vi "domeADB_getEvent_BrakeEngaged.vi"(8 "error in (no error)":errorcluster, 11 "logevent_BrakeEngaged_Ctl":T1) -> (0 "error out":errorcluster, 2 "function return":i32, 3 "logevent_BrakeEngaged_Ctl out":T1)   [LabVIEW 2016, in "SALLV_domeADB.lvlib"]
doc: "int domeADB_shm_getEvent_BrakeEngagedLV(domeADB_logevent_BrakeEngagedLV *logevent_BrakeEngaged_Ctl );"
uses:
  SALLV_domeADB.lvlib
  DataTypes/logevent_BrakeEngaged.ctl
  SALLV_domeADB.so
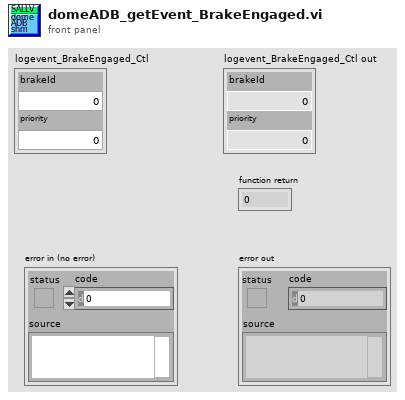
[diagram p1: front panel]
types:
  T1 = typedef "SALLV_domeADB.lvlib/logevent_BrakeEngaged.ctl" = cluster{"brakeId":i32, "priority":i32}
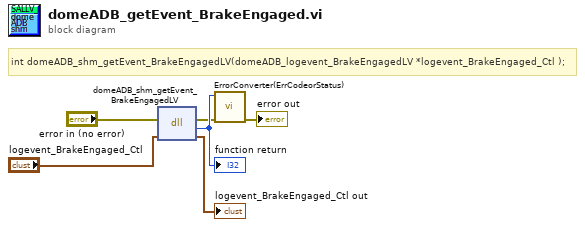
[diagram p0: block diagram]
diagram:
  # "int domeADB_shm_getEvent_BrakeEngagedLV(domeADB_logevent_BrakeEngagedLV *logevent_BrakeEngaged_Ctl );"
  n1 = dll-call lib="home/andres/Desktop/SALLV_domeADB/SALLV_domeADB.*" fn="domeADB_shm_getEvent_BrakeEngagedLV"(error in="error in (no error)", "logevent_BrakeEngaged_Ctl"="logevent_BrakeEngaged_Ctl") -> (error out=w2:errorcluster, w6:i32, "logevent_BrakeEngaged_Ctl"=→"logevent_BrakeEngaged_Ctl out":T1)  [unwired: 2 in, 1 out]
  "function return" <- w6
  n2 = call "ErrorConverter(ErrCodeorStatus).vi"("error in (no error)"=w2, "error code"=w6) -> ("error out"=→"error out":errorcluster)  [unwired: 9 in]
